vi "Unbundle.vi"(8 "error in (no error)":errorcluster, 11 "Multi Instrument Handler in":refnum<class "Multi Instrument Handler.lvclass">) -> (0 "error out":errorcluster, 1 "Hander Index":i32, 2 "Aquirer Lock":T1, 3 "Multi Instrument Handler out":refnum<class "Multi Instrument Handler.lvclass">, 4 "Caller Enqueuer":refnum<class "Message Enqueuer.lvclass">, 5 "Aquisition queue":refnum<queue>)   [LabVIEW 2020, in "Instrument Handler.lvlib" / "Multi Instrument Handler.lvclass"]
doc: "Read the private data of the Multi Instrument Handler as well as the Caller Enqueuer."
uses:
  Multi Instrument Handler.lvclass
  C:/Current projects/WS/PPL/HDH.Actor Framework.Core.Actor.lvlibp/1abvi3w/vi.lib/ActorFramework/Actor/Actor.lvclass
  Controls/Ctl_AquirerCompletionStatus.ctl
  PPL/HDH.Actor Framework.Core.Actor.lvlibp/1abvi3w/vi.lib/ActorFramework/Message Enqueuer/Message Enqueuer.lvclass
  Multi Instrument Handler.lvclass/Multi Instrument Handler.ctl
  PPL/HDH.Actor Framework.Core.Actor.lvlibp/1abvi3w/vi.lib/ActorFramework/Actor/Actor.lvclass
  Instrument Handler.lvlib
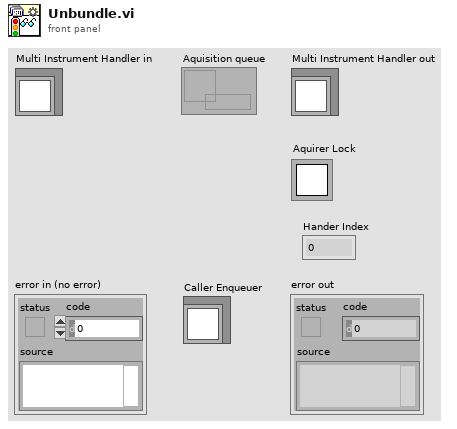
[diagram p1: front panel]
types:
  T1 = typedef "Semaphore RefNum" = refnum<k1>
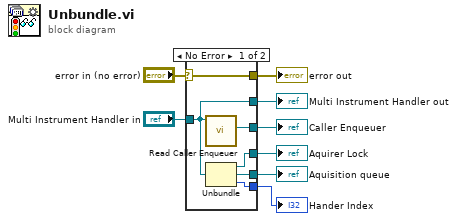
[diagram p0: block diagram]
diagram:
  n1 = case shown="No Error" "error in (no error)" {
    selector: "error in (no error)" -> [w14 w15]
    tunnel: [w14 w15] -> w7
    tunnel: [w10 w16] -> w5
    tunnel: "Multi Instrument Handler in" -> [w10 w16]
    tunnel: [w13 _] -> w4
    tunnel: [w12 _] -> w3
    tunnel: [w11 _] -> w2
    tunnel: [w9 _] -> w1
    frame No Error {
      n2 = call "Read Caller Enqueuer.vi"("Actor"=w10) -> ("Caller Enqueuer"=w9:refnum<class "Message Enqueuer.lvclass">)  [unwired: 10 in]
      n3 = Unbundle(w10) -> (w13:T1, w11:refnum<queue>, w12:i32)
    }
    frame Error {
    }
  }
  "error out" <- w7
  "Multi Instrument Handler out" <- w5
  "Aquirer Lock" <- w4
  "Hander Index" <- w3
  "Aquisition queue" <- w2
  "Caller Enqueuer" <- w1
